vi "Stand Alone Test for Find Complete Frame.vi"() -> ()   [LabVIEW 2017]
uses:
  Libraries/iTacho_class/iTacho.lvclass
panel:
  out "Test Pass?":bool
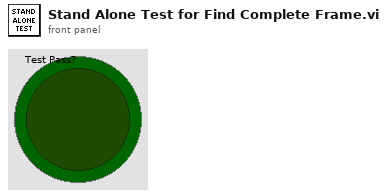
[diagram p1: front panel]
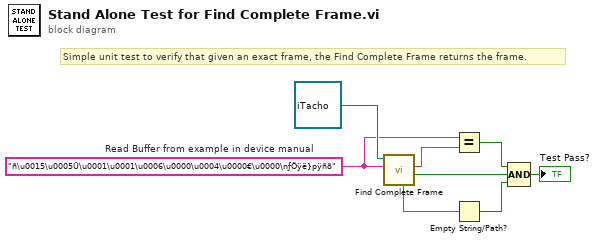
[diagram p0: block diagram]
diagram:
  w5 = "ñ\u0015\u0005Ü\u0001\u0001\u0006\u0000\u0004\u0000€\u0000\nƒÖÿë}pÿñõ"  # Read Buffer from example in device manual
  # "Simple unit test to verify that given an exact frame, the Find Complete Frame returns the frame."
  n1 = call-dynamic "Find Complete Frame.vi"("Read Buffer in"=w5, "iTacho in"=refnum<class "iTacho.lvclass"> refnum) -> ("Found New Frame?"=w7:bool, "Frame"=w6:string, "Left Over Bytes"=w3:string)  [unwired: 5 in, 2 out]
  n2 = Equal?(x=w5, y=w6) -> (x = y?=w4:bool)
  n3 = Empty String/Path?(string/path=w3) -> (empty?=w2:bool)
  n4 = Compound Arithmetic op=AND(w4, w7, w2) -> (→"Test Pass?":bool)
